vi "Examen_03_Proyecto.vi"() -> ()   [LabVIEW 2020]
uses:
  <vilib>/Instr/_visa.llb/VISA Configure Serial Port (Instr).vi
panel:
  out "Temperatura 2":dbl
  in  "write buffer 2":string
  in  "Ingresar Temperatura":dbl
  in  "Modo manual":bool
  out "Temperatura DAQ":dbl
  in  "Stop Button":bool
  out "Numeric":i32
  in  "VISA resource name":refnum<visa-resource-name>
  # "APARADOR POR ESTACIONES"
  # "MODO AUTOMATICO"
  # "MODO MANUAL"
  # "TEMPERATURA REGISTRADA"
  # "INGRESA LA TEMPERATURA DESEADA"
  # "INVIERNO        <=10°"
  # "OTOÑO              10°>X >=18"
  # "TEMPERATURA REGISTRADA"
  # "PRIMAVERA  18°>X >=24°"
  # "PARA CAMBIAR A MODO MANUAL\nPRESIONAR EL SIGUIENTE BOTON"
  # "VERANO          > 24°"
  # "PUERTO COM"
  # "DATO ENVIADO"
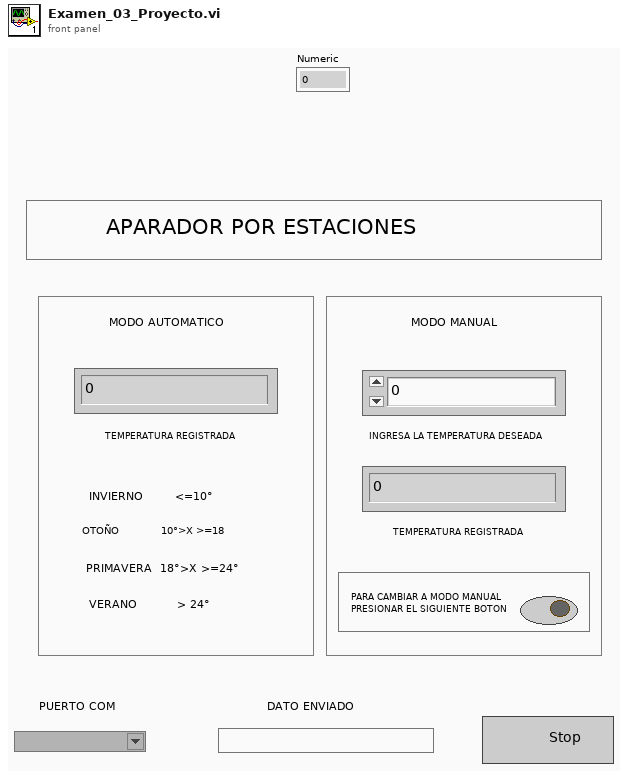
[diagram p1: front panel]
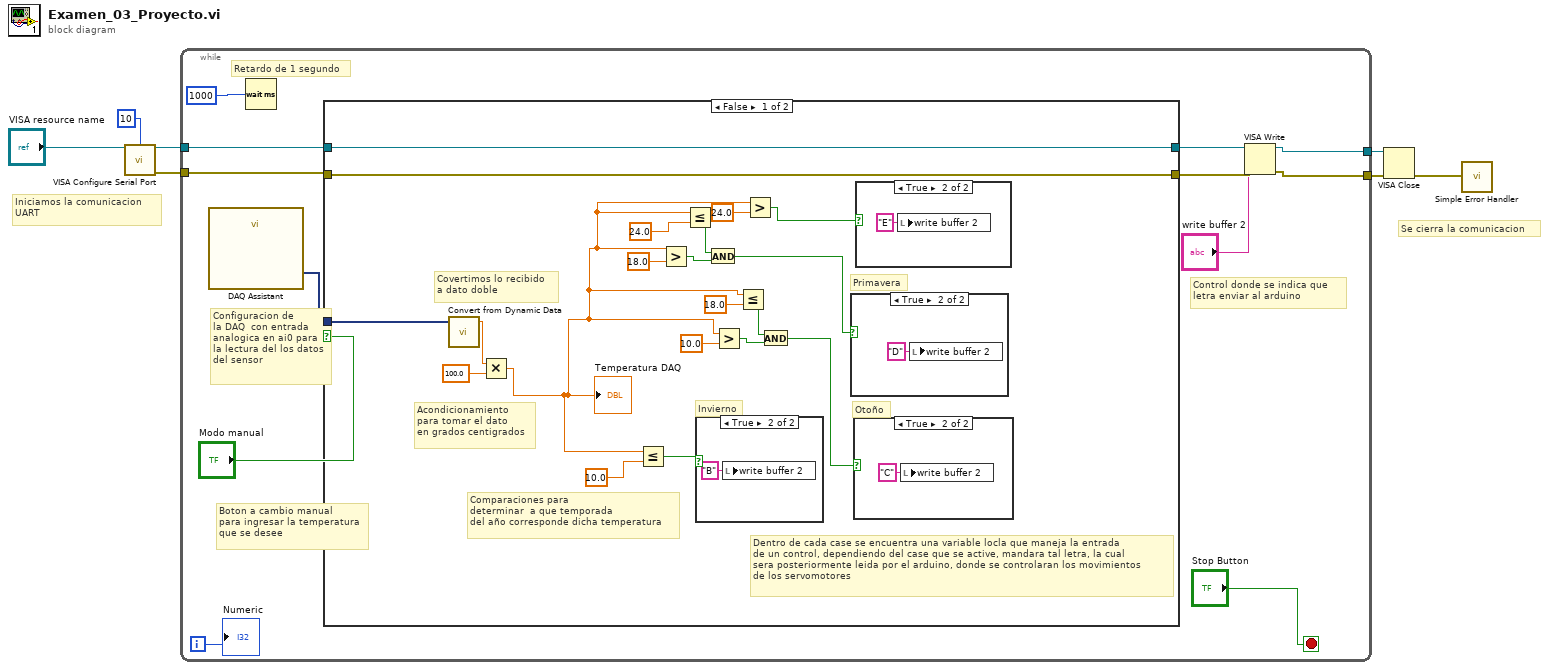
[diagram p0: block diagram]
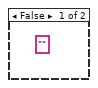
[diagram p5: hidden frame]
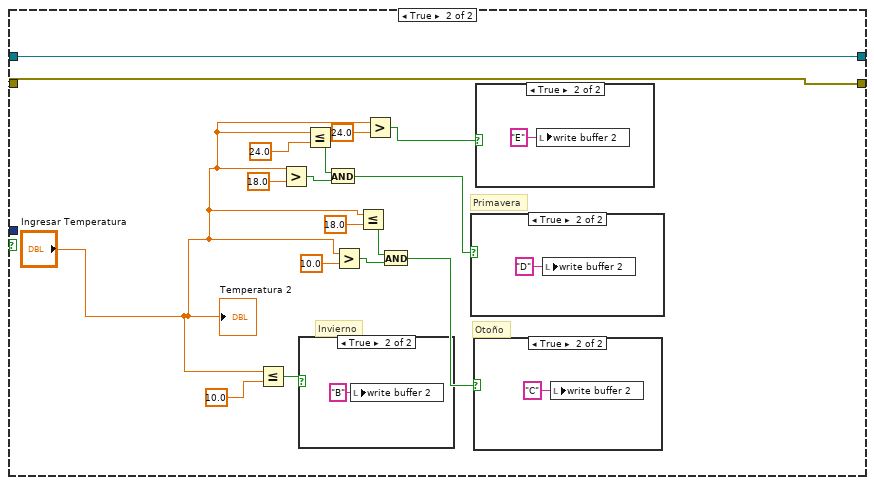
[diagram p6: hidden frame]
diagram:
  # "Se cierra la comunicacion"
  # "Iniciamos la comunicacion \nUART"
  n1 = call-poly "VISA Configure Serial Port"("VISA resource name"="VISA resource name", "termination char\n(0xA = '\\n' = LF)"=u8 10 ("termination char\n(0xA = '\\n' = LF)")) -> ("VISA resource name out"=w5:refnum<visa-resource-name>, "error out"=w4:errorcluster)  [unwired: 12 in]
  n2 = while {
    tunnel: w5 -> [w14]
    tunnel: w4 -> [w13]
    tunnel: [w18] -> w2
    tunnel: [w17] -> w1
    i -> [w11]
    stop <- "Stop Button" stop-if-true
    # "Control donde se indica que \nletra enviar al arduino"
    # "Boton a cambio manual\npara ingresar la temperatura\nque se desee"
    # "Configuracion de\nla DAQ  con entrada\nanalogica en ai0 para\nla lectura del los datos\ndel sensor"
    # "Retardo de 1 segundo"
    n3 = call "DAQ Assistant"() -> ("data"=w8:dynamicdata)  [unwired: 17 in, 2 out]
    n4 = Wait (ms)(milliseconds to wait=u32 1000) -> ()  [unwired: 1 out]
    n5 = case shown="False" "Modo manual" {
      tunnel: w14 -> [w24 w45]
      tunnel: w13 -> [w23 w44]
      tunnel: [w24 w45] -> w16
      tunnel: [w23 w44] -> w15
      tunnel: w8 -> [w20 _]
      frame False {
        # "Dentro de cada case se encuentra una variable locla que maneja la entrada\nde un control, dependiendo del case que se active, mandara tal letra, la cual \nsera posteriormente leida por el arduino, donde se controlaran los movimientos\nde los servomotores"
        # "Comparaciones para \ndeterminar  a que temporada\ndel año corresponde dicha temperatura"
        # "Acondicionamiento\npara tomar el dato \nen grados centigrados"
        # "Covertimos lo recibido\na dato doble"
        # "Primavera"
        # "Otoño"
        # "Invierno"
        n6 = call "Convert from Dynamic Data"("Dynamic Data Type"=w20) -> ("Scalar"=w22:dbl)  [unwired: 3 in]
        n7 = Multiply(x=w22, y=100.0) -> (x*y=w21:dbl)
        "Temperatura DAQ" <- w21
        n8 = Less Or Equal?(x=w21, y=10.0) -> (x <= y?=w37:bool)
        n9 = Greater?(x=w21, y=18.0) -> (0:w29:bool)
        n10 = Less Or Equal?(x=w21, y=24.0) -> (x <= y?=w30:bool)
        n11 = case shown="True" w37 {
          frame False {
            (unwired) ""
          }
          frame True {
            n12 = local write "write buffer 2"("B" ("write buffer")) -> ()
          }
        }
        n13 = And(x=w30, y=w29) -> (x .and. y?=w27:bool)
        n14 = Greater?(x=w21, y=10.0) -> (0:w35:bool)
        n15 = Less Or Equal?(x=w21, y=18.0) -> (x <= y?=w34:bool)
        n16 = Greater?(x=w21, y=24.0) -> (0:w25:bool)
        n17 = And(x=w34, y=w35) -> (x .and. y?=w32:bool)
        n18 = case shown="True" w27 {
          frame False {
          }
          frame True {
            n19 = local write "write buffer 2"("D" ("write buffer")) -> ()
          }
        }
        n20 = case shown="True" w32 {
          frame False {
          }
          frame True {
            n21 = local write "write buffer 2"("C" ("write buffer")) -> ()
          }
        }
        n22 = case shown="True" w25 {
          frame False {
          }
          frame True {
            n23 = local write "write buffer 2"("E" ("write buffer")) -> ()
          }
        }
      }
      frame True {
        # "Primavera"
        # "Otoño"
        # "Invierno"
        n24 = Less Or Equal?(x="Ingresar Temperatura", y=10.0) -> (x <= y?=w59:bool)
        n25 = Greater?(x="Ingresar Temperatura", y=18.0) -> (0:w51:bool)
        n26 = case shown="True" w59 {
          frame False {
          }
          frame True {
            n27 = local write "write buffer 2"("B" ("write buffer")) -> ()
          }
        }
        n28 = Less Or Equal?(x="Ingresar Temperatura", y=24.0) -> (x <= y?=w52:bool)
        n29 = And(x=w52, y=w51) -> (x .and. y?=w49:bool)
        n30 = Greater?(x="Ingresar Temperatura", y=10.0) -> (0:w57:bool)
        n31 = Less Or Equal?(x="Ingresar Temperatura", y=18.0) -> (x <= y?=w56:bool)
        n32 = Greater?(x="Ingresar Temperatura", y=24.0) -> (0:w47:bool)
        n33 = And(x=w56, y=w57) -> (x .and. y?=w54:bool)
        n34 = case shown="True" w49 {
          frame False {
          }
          frame True {
            n35 = local write "write buffer 2"("D" ("write buffer 2")) -> ()
          }
        }
        n36 = case shown="True" w54 {
          frame False {
          }
          frame True {
            n37 = local write "write buffer 2"("C" ("write buffer 2")) -> ()
          }
        }
        n38 = case shown="True" w47 {
          frame False {
          }
          frame True {
            n39 = local write "write buffer 2"("E" ("write buffer 2")) -> ()
          }
        }
        "Temperatura 2" <- "Ingresar Temperatura"
      }
    }
    n40 = VISA Write(VISA resource name=w16, write buffer="write buffer 2", error in (no error)=w15) -> (VISA resource name out=w18:refnum<visa-resource-name>, error out=w17:errorcluster)  [unwired: 1 out]
    "Numeric" <- w11
  }
  n41 = VISA Close(VISA resource name=w2, error in (no error)=w1) -> (error out=w3:errorcluster)
  n42 = call <vilib>:"Simple Error Handler.vi"("error in (no error)"=w3) -> ()  [unwired: 4 in, 5 out]
